vi "Delay PanelUpdata.vi"(8 "error in (no error)":errorcluster caption="错误输入（无错误）", 10 "延迟前面板更新":bool, 11 "PanelRootNode 输入":refnum<class "PanelRootNode.lvclass"> caption="DNL_LabVIEW Object in") -> (0 "error out":errorcluster caption="错误输出", 3 "PanelRootNode 输出":refnum<class "PanelRootNode.lvclass"> caption="DNL_LabVIEW Object out")   [LabVIEW 2013, in "PanelRootNode.lvclass"]
uses:
  PanelRootNode.lvclass
  PanelRootNode.lvclass/PanelRootNode.ctl
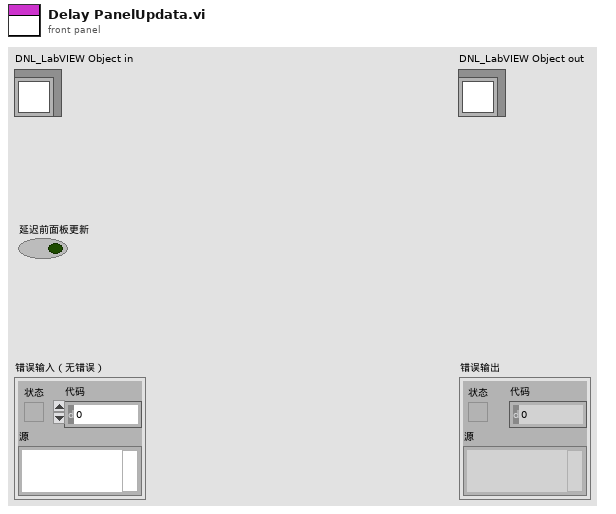
[diagram p1: front panel]
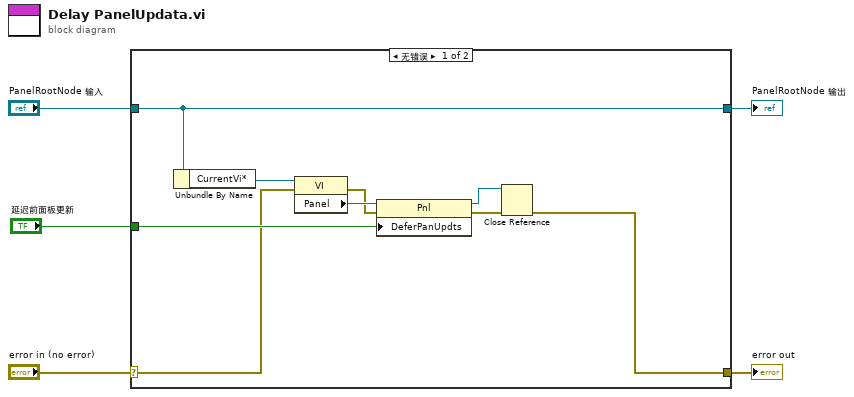
[diagram p0: block diagram]
diagram:
  n1 = case shown="无错误" "error in (no error)" {
    selector: "error in (no error)" -> [w9 w16]
    tunnel: [w7 w16] -> w4
    tunnel: [w14 w15] -> w2
    tunnel: "PanelRootNode 输入" -> [w14 w15]
    tunnel: "延迟前面板更新" -> [w11 _]
    frame No Error {
      n2 = Unbundle By Name(w14) -> ("CurrentVi*"=w13:refnum<vi>)
      n3 = property class="VI"(reference=w13, error in=w9) -> (error out=w10:errorcluster, "Panel"=w12:refnum<vi>)  [unwired: 1 out]
      n4 = property class="Pnl"(reference=w12, error in=w10, "DeferPanUpdts"=w11) -> (reference out=w6:refnum<vi>, error out=w8:errorcluster)
      n5 = Close Reference(reference=w6, error in (no error)=w8) -> (error out=w7:errorcluster)
    }
    frame Error {
    }
  }
  "error out" <- w4
  "PanelRootNode 输出" <- w2
